vi "Loop Counter With Reset.vi"(10 "Max Count":u32, 11 "Enable/nReset":bool) -> (2 "Count":u32, 3 "Count Triggered":bool)   [LabVIEW 2017]
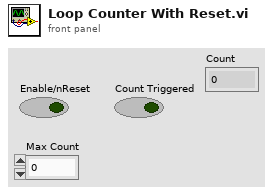
[diagram p1: front panel]
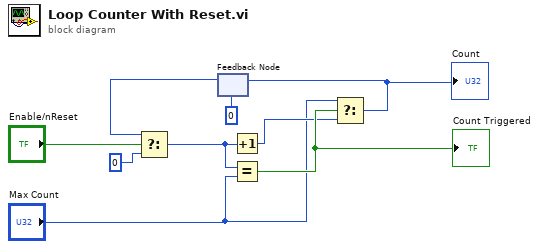
[diagram p0: block diagram]
diagram:
  n1 = feedback #1(u32 0 ("initial value 2")) -> (w9:u32)
  n2 = Select ("Select 2")(t=w9, s="Enable/nReset", f=u32 0) -> (s? t:f=w1:u32)
  n3 = Increment(x=w1) -> (x+1=w4:u32)
  n4 = Equal?(x=w1, y="Max Count") -> (x = y?=w5:bool)
  "Count Triggered" <- w5
  n5 = Select(t="Max Count", s=w5, f=w4) -> (s? t:f=w2:u32)
  "Count" <- w2
  n6 = feedback-in #1 ("2")(w2) -> ()
